vi "dds reader config to writer.vi"(11 "reader configuration":T2) -> (3 "writer configuration":T1)   [LabVIEW 2020, in "DDS configuration.lvclass"]
uses:
  dds configuration.lvclass
  <vilib>/RTI DDS Toolkit/Types/RTI DDS Advanced Reader Configuration.ctl
  <vilib>/RTI DDS Toolkit/Types/RTI DDS Advanced Writer Configuration.ctl
  <vilib>/RTI DDS Toolkit/Library/LVDDS_library.lvlib
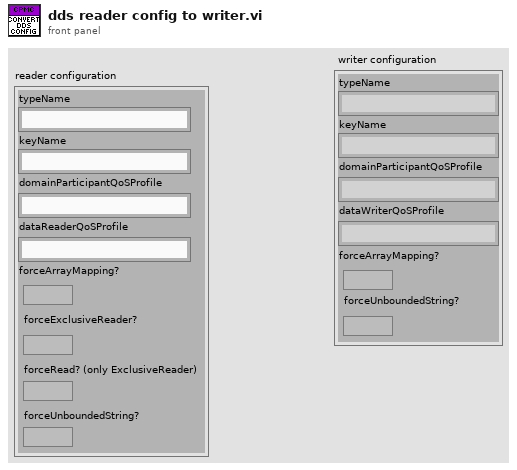
[diagram p1: front panel]
types:
  T1 = typedef "LVDDS_library.lvlib/RTI DDS Advanced Writer Configuration.ctl" = cluster{"typeName":string, "keyName":string, "domainParticipantQoSProfile":string, "dataWriterQoSProfile":string, "forceArrayMapping?":bool, "forceUnboundedString?":bool}
  T2 = typedef "LVDDS_library.lvlib/RTI DDS Advanced Reader Configuration.ctl" = cluster{"typeName":string, "keyName":string, "domainParticipantQoSProfile":string, "dataReaderQoSProfile":string, "forceArrayMapping?":bool, "forceExclusiveReader?":bool, "forceRead? (only ExclusiveReader)":bool, "forceUnboundedString?":bool}
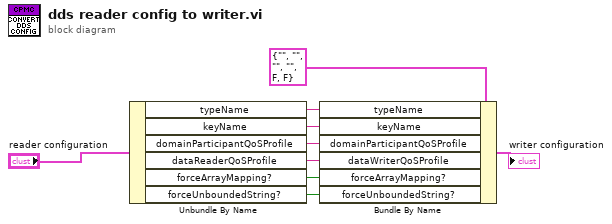
[diagram p0: block diagram]
diagram:
  n1 = Unbundle By Name("reader configuration") -> ("typeName"=w6:string, "keyName"=w5:string, "domainParticipantQoSProfile"=w4:string, "dataReaderQoSProfile"=w3:string, "forceArrayMapping?"=w2:bool, "forceUnboundedString?"=w1:bool)
  n2 = Bundle By Name(cluster=T1 {"typeName"="", "keyName"="", "domainParticipantQoSProfile"="", "dataWriterQoSProfile"="", "forceArrayMapping?"=FALSE, "forceUnboundedString?"=FALSE} ("writer configuration"), "typeName"=w6, "keyName"=w5, "domainParticipantQoSProfile"=w4, "dataWriterQoSProfile"=w3, "forceArrayMapping?"=w2, "forceUnboundedString?"=w1) -> (→"writer configuration":T1)
